vi "ones.vi"   [LabVIEW 2014, in "NI_Gmath.lvlib"]
uses:
  NI_Gmath.lvlib
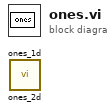
[diagram p0: block diagram]
diagram:
  n1 = call "ones_2d.vi"() -> ()  [unwired: 8 in, 1 out]
  n2 = call "ones_1d.vi"() -> ()  [unwired: 8 in, 1 out]
